vi "ReadAllAdv.vi"(4 "TypeMap in":refnum<class "TypeMap.lvclass">, 5 "Select *":bool=TRUE, 6 "commandTimeout":i32, 7 "Where":string, 8 "error in (no error)":errorcluster, 9 "ReadCfg":T1, 10 "object in":refnum<class>, 11 "SqlMapper in":refnum<class "SqlMapper.lvclass">) -> (0 "error out":errorcluster, 2 "Query Result out":refnum<class "Query Result.lvclass">, 3 "SqlMapper out":refnum<class "SqlMapper.lvclass">)   [LabVIEW 2020, in "ORM.lvlib" / "TypeMap.lvclass"]
uses:
  TypeMap.lvclass
  TypeMap.lvclass/TypeMap.ctl
  SqlMapper/SqlMapper.lvclass
  Query Result/Query Result.lvclass
  DbConnection/OrderBy.ctl
  ORM.lvlib
  DbConnection/AdvReadCfg.ctl
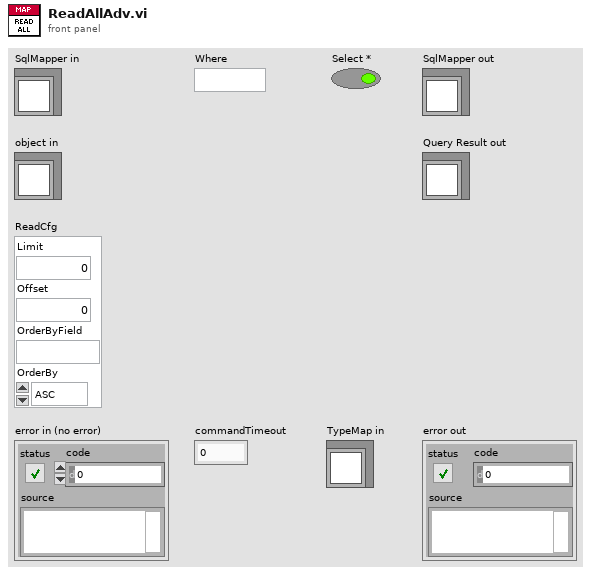
[diagram p1: front panel]
types:
  T1 = typedef "ORM.lvlib/AdvReadCfg.ctl" = cluster{"Limit":i64, "Offset":i64, "OrderByField":string, "OrderBy":T2}
  T2 = typedef "ORM.lvlib/OrderBy.ctl" = enum16{"ASC", "DESC"}
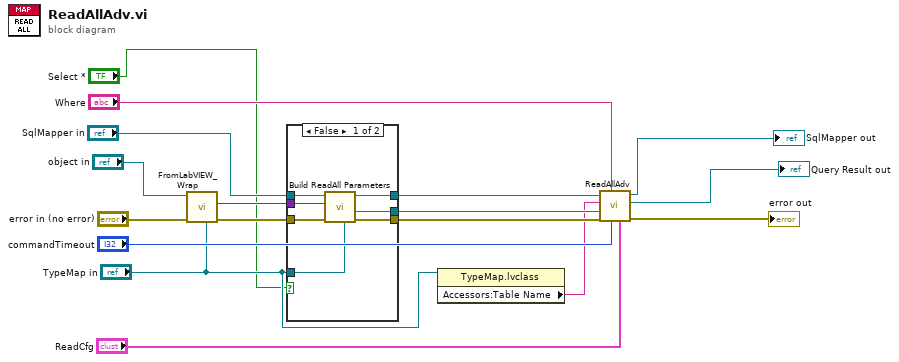
[diagram p0: block diagram]
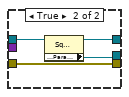
[diagram p2: hidden frame]
diagram:
  n1 = call "FromLabVIEW_Wrap.vi"("TypeMap in"="TypeMap in", "error in (no error)"="error in (no error)", "object in"="object in") -> ("error out"=w14:errorcluster, "DbRow"=w15:variant)  [unwired: 7 in]
  n2 = case shown="False" "Select *" {
    tunnel: "SqlMapper in" -> [w24 w28]
    tunnel: w15 -> [w23 _]
    tunnel: w14 -> [w22 w27]
    tunnel: [w21 w27] -> w11
    tunnel: [w20 w26] -> w10
    tunnel: [w19 w25] -> w8
    tunnel: "TypeMap in" -> [w18 _]
    frame False {
      n3 = call-dynamic "Build ReadAll Parameters.vi"("TypeMap in"=w18, "error in (no error)"=w22, "object"=w23, "SqlMapper in"=w24) -> ("error out"=w21:errorcluster, "DynamicParameters out"=w19:refnum<class "DynamicParameters.lvclass">, "SqlMapper out"=w20:refnum<class "SqlMapper.lvclass">)  [unwired: 5 in]
    }
    frame True {
      n4 = property class="SqlMapper.lvclass"(reference=w28) -> (reference out=w26:refnum<class "SqlMapper.lvclass">, "Accessors:Parameter"=w25:refnum<class "DynamicParameters.lvclass">)  [unwired: 1 in, 1 out]
    }
  }
  n5 = property class="TypeMap.lvclass"(reference="TypeMap in") -> ("Accessors:Table Name"=w6:string)  [unwired: 1 in, 2 out]
  n6 = call "ReadAllAdv.vi"("ReadCfg"="ReadCfg", "commandTimeout"="commandTimeout", "Where"="Where", "error in (no error)"=w11, "DynamicParameters"=w8, "TableName"=w6, "SqlMapper in"=w10) -> ("error out"=→"error out":errorcluster, "Query Result out"=→"Query Result out":refnum<class "Query Result.lvclass">, "SqlMapper out"=→"SqlMapper out":refnum<class "SqlMapper.lvclass">)  [unwired: 2 in]
